vi "Power Source Settings.vi"(8 "error in":errorcluster, 9 "volt":dbl=14.0 format="%#_13g", 10 "Action":T1(ring), 11 "COM":refnum<visa-resource-name>="COM3") -> (0 "error out":errorcluster, 3 "read buffer":string)   [LabVIEW 2014]
uses:
  <vilib>/Instr/_visa.llb/VISA Configure Serial Port (Instr).vi
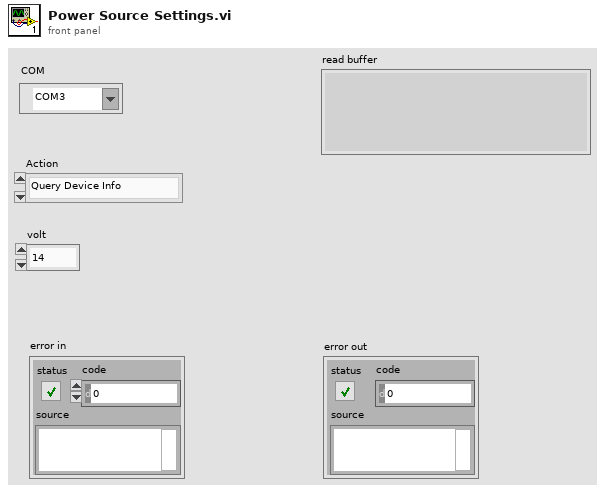
[diagram p1: front panel]
types:
  T1 = enum16{"Query Device Info", "Set Voltage", "Read Voltage", "Set Current", "Read Current", "Enable Output", "Disable Output", "Set to Remote", "Set to Local", "Get Errors", "Set Protect Voltage", "Read Protect Voltage"}
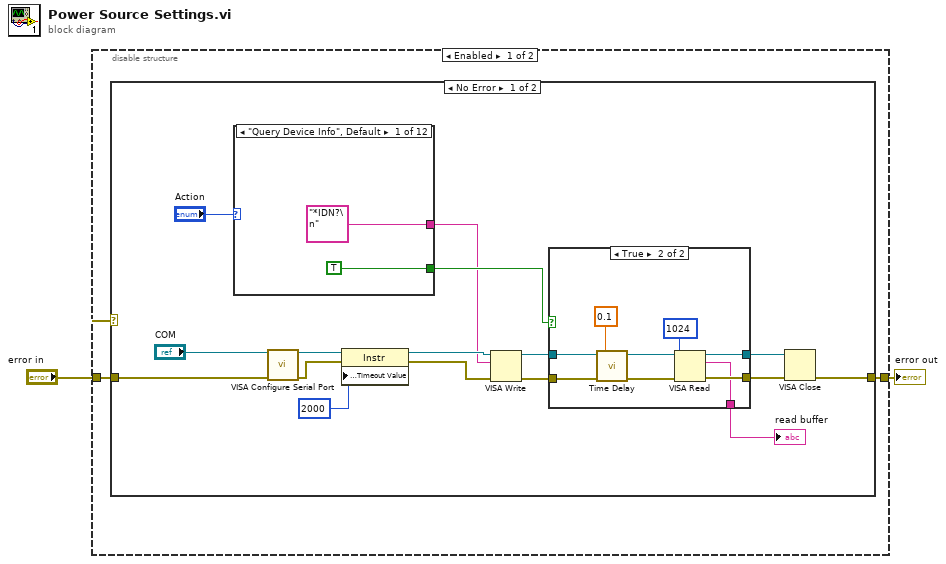
[diagram p0: block diagram]
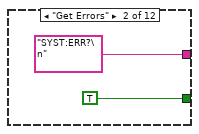
[diagram p2: hidden frame]
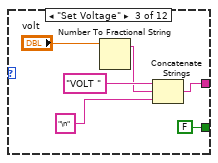
[diagram p3: hidden frame]
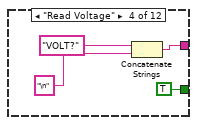
[diagram p4: hidden frame]
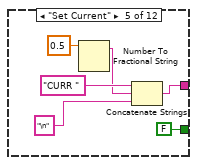
[diagram p5: hidden frame]
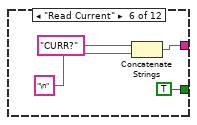
[diagram p6: hidden frame]
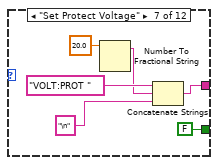
[diagram p7: hidden frame]
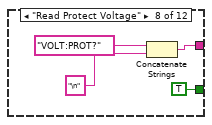
[diagram p8: hidden frame]
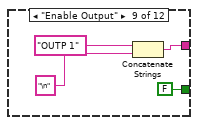
[diagram p9: hidden frame]
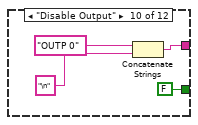
[diagram p10: hidden frame]
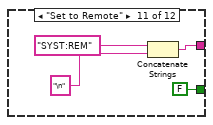
[diagram p11: hidden frame]
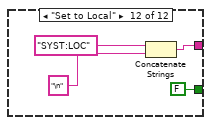
[diagram p12: hidden frame]
diagram:
  n1 = disable-structure shown="Enabled" {
    disable-tunnel: [w4 w82] -> w2
    disable-tunnel: "error in" -> [w3 w82]
    frame Enabled {
      n2 = case shown="No Error" w3 {
        tunnel: [w12 w81] -> w4
        tunnel: w3 -> [w8 w81]
        frame No Error {
          n3 = case shown="\"Query Device Info\", Default" "Action" {
            tunnel: [TRUE TRUE FALSE TRUE FALSE TRUE FALSE TRUE FALSE FALSE FALSE FALSE] -> w6
            tunnel: ["*IDN?\n" ("Command") "SYST:ERR?\n" ("Command") w27 w32 w37 w42 w47 w52 w56 w60 w64 w68] -> w5
            frame "Query Device Info", Default {
            }
            frame "Get Errors" {
            }
            frame "Set Voltage" {
              n4 = Number To Fractional String(number="volt") -> (F-format string=w29:string)  [unwired: 3 in]
              n5 = Concatenate Strings("VOLT " ("Command"), w29, "\n") -> (w27:string)
            }
            frame "Read Voltage" {
              n6 = Concatenate Strings("VOLT?" ("Command"), "\n") -> (w32:string)
            }
            frame "Set Current" {
              n7 = Number To Fractional String(number=0.5) -> (F-format string=w39:string)  [unwired: 3 in]
              n8 = Concatenate Strings("CURR " ("Command"), w39, "\n") -> (w37:string)
            }
            frame "Read Current" {
              n9 = Concatenate Strings("CURR?" ("Command"), "\n") -> (w42:string)
            }
            frame "Set Protect Voltage" {
              n10 = Number To Fractional String(number=20.0) -> (F-format string=w49:string)  [unwired: 3 in]
              n11 = Concatenate Strings("VOLT:PROT " ("Command"), w49, "\n") -> (w47:string)
            }
            frame "Read Protect Voltage" {
              n12 = Concatenate Strings("VOLT:PROT?" ("Command"), "\n") -> (w52:string)
            }
            frame "Enable Output" {
              n13 = Concatenate Strings("OUTP 1" ("Command"), "\n") -> (w56:string)
            }
            frame "Disable Output" {
              n14 = Concatenate Strings("OUTP 0" ("Command"), "\n") -> (w60:string)
            }
            frame "Set to Remote" {
              n15 = Concatenate Strings("SYST:REM" ("Command"), "\n") -> (w64:string)
            }
            frame "Set to Local" {
              n16 = Concatenate Strings("SYST:LOC" ("Command"), "\n") -> (w68:string)
            }
          }
          n17 = call-poly "VISA Configure Serial Port"("VISA resource name"="COM", "error in (no error)"=w8) -> ("VISA resource name out"=w14:refnum<visa-resource-name>, "error out"=w10:errorcluster)  [unwired: 12 in]
          n18 = property class="Instr"(reference=w14, error in=w10, "General Settings:Timeout Value"=u32 2000) -> (reference out=w13:refnum<visa-resource-name>, error out=w11:errorcluster)
          n19 = VISA Write(VISA resource name=w13, write buffer=w5, error in (no error)=w11) -> (VISA resource name out=w9:refnum<visa-resource-name>, error out=w20:errorcluster)  [unwired: 1 out]
          n20 = case shown="True" w6 {
            tunnel: w20 -> [w71 w80]
            tunnel: [w71 w79] -> w19
            tunnel: [w72 w78] -> w18
            tunnel: [_ w77] -> w17
            tunnel: w9 -> [w72 w73]
            frame False {
            }
            frame True {
              n21 = call "Time Delay"("error in (no error)"=w80, "Delay Time (s)"=0.1) -> ("error out"=w75:errorcluster)  [unwired: 9 in]
              n22 = VISA Read(VISA resource name=w73, byte count=u32 1024, error in (no error)=w75) -> (VISA resource name out=w78:refnum<visa-resource-name>, read buffer=w77:string, error out=w79:errorcluster)  [unwired: 1 out]
            }
          }
          "read buffer" <- w17
          n23 = VISA Close(VISA resource name=w18, error in (no error)=w19) -> (error out=w12:errorcluster)
        }
        frame Error {
        }
      }
    }
    frame Disabled {
    }
  }
  "error out" <- w2
